vi "oa_Check DC Gap Input Data (N Channels).vi"(0 "even angle signals":cluster{"r0":dbl, "dr":dbl, "Y":dbl[]}[](array[cluster]) {"r0" format="%.2p"; "dr" format="%.2p"; "Y" format="%.2f"}, 1 "reset?":bool=TRUE, 5 "DC gap references [V]":dbl[](array[numeric]), 7 "averaging type in":enum16{"Linear", "Exponential"}(ring), 9 "window in":T1(ring), 11 "error in (no error)":errorcluster) -> (2 "reset DC ref?":bool, 3 "reset out?":bool, 4 "even angle signals":cluster{"r0":dbl, "dr":dbl, "Y":dbl[]}[](array[cluster]) {"r0" format="%.2p"; "dr" format="%.2p"; "Y" format="%.2f"}, 6 "DC gap reference [V]":dbl[](array[numeric]), 8 "averaging type":enum16{"Linear", "Exponential"}(ring), 10 "window":T1(ring), 15 "error out":errorcluster)   [LabVIEW 2017, in "SoundVib_RefDataProcess.lvlib"]
uses:
  <vilib>/addons/Sound and Vibration/Order Analysis/Referece Data Processing/SoundVib_RefDataProcess.lvlib
  <vilib>/addons/Sound and Vibration/Order Analysis/Resample Order Tracking/SubVIs/OAT Verify Resampled Signal (Multi Channels).vi
  <vilib>/addons/Sound and Vibration/Order Analysis/Resample Order Tracking/SoundVib_Resampling.lvlib
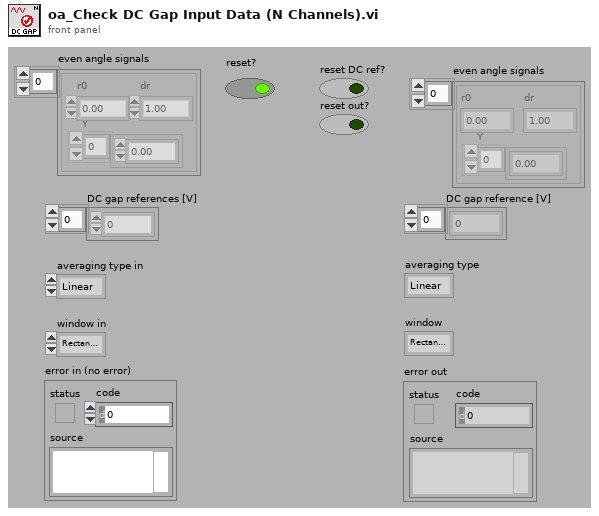
[diagram p1: front panel]
types:
  T1 = enum16{"Rectangular (none)", "Hanning", "Low side lobe"}
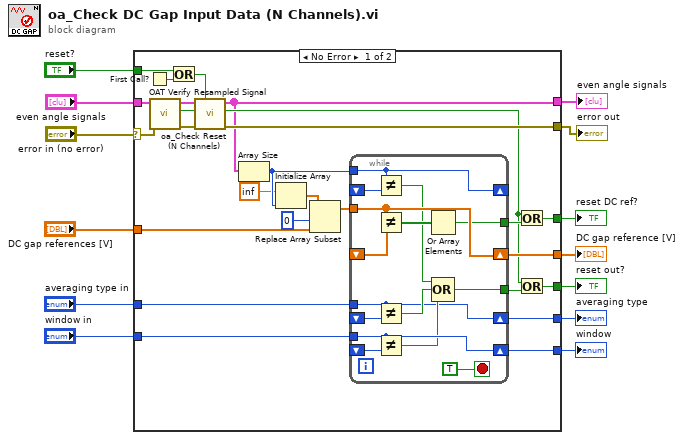
[diagram p0: block diagram]
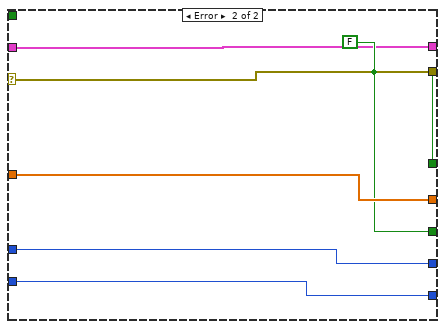
[diagram p2: hidden frame]
diagram:
  n1 = case shown="No Error" "error in (no error)" {
    selector: "error in (no error)" -> [w25 w58]
    tunnel: [w29 w56] -> w13
    tunnel: [w39 w59] -> w12
    tunnel: [w38 w60] -> w11
    tunnel: [w27 w56] -> w10
    tunnel: [w37 w57] -> w9
    tunnel: "DC gap references [V]" -> [w34 w57]
    tunnel: "window in" -> [w36 w59]
    tunnel: "averaging type in" -> [w35 w60]
    tunnel: "even angle signals" -> [w26 w55]
    tunnel: [w16 w58] -> w4
    tunnel: [w14 w55] -> w2
    tunnel: "reset?" -> [w31 _]
    frame No Error {
      n2 = First Call?() -> (First Call?: T/F=w32:bool)
      n3 = call-poly <vilib>:"OAT Verify Resampled Signal.vi"("error in (no error)"=w25, "resampled signal"=w26) -> ("error out"=w17:errorcluster, "empty signal"=w18:bool, "resampled signal out"=w20:cluster{"r0":dbl, "dr":dbl, "Y":dbl[]}[])  [unwired: 7 in]
      n4 = Or(x=w31, y=w32) -> (x .or. y?=w19:bool)
      n5 = call <vilib>:"oa_Check Reset (N Channels).vi"("reset?"=w19, "error in (no error)"=w17, "empty?"=w18, "resampled signal"=w20) -> ("error out"=w16:errorcluster, "reset?"=w15:bool, "resampled signal out"=w14:cluster{"r0":dbl, "dr":dbl, "Y":dbl[]}[])  [unwired: 5 in]
      n6 = Array Size(array=w14) -> (size(s)=w33:i32)
      n7 = Initialize Array(inf ("element"), w33) -> (w23:dbl[])
      n8 = Replace Array Subset(array=w23, new element=w34, index=0) -> (w22:dbl[])
      n9 = while {
        tunnel: w35 -> [w47]
        tunnel: w36 -> [w51]
        shift-right: [w47] -> w38
        shift-left: _ -> [w53]
        shift-right: [w51] -> w39
        shift-left: _ -> [w52]
        tunnel: [w48] -> w28
        tunnel: w22 -> [w44]
        shift-right: [w44] -> w37
        shift-left: _ -> [w46]
        tunnel: [w41] -> w30
        tunnel: w33 -> [w42]
        shift-right: [w42] -> _
        shift-left: _ -> [w43]
        stop <- TRUE stop-if-true
        n10 = Not Equal?(x=w42, y=w43) -> (x != y?=w40:bool)
        n11 = Not Equal?(x=w44, y=w46) -> (x != y?=w45:bool[])
        n12 = Not Equal?(x=w47, y=w53) -> (x != y?=w50:bool)
        n13 = Not Equal?(x=w51, y=w52) -> (x != y?=w49:bool)
        n14 = Or Array Elements(Boolean array=w45) -> (logical OR=w41:bool)
        n15 = Compound Arithmetic op=OR(w40, w50, w49) -> (w48:bool)
      }
      n16 = Or(x=w15, y=w30) -> (x .or. y?=w29:bool)
      n17 = Or(x=w15, y=w28) -> (x .or. y?=w27:bool)
    }
    frame Error {
      w56 = FALSE
    }
  }
  "reset DC ref?" <- w13
  "window" <- w12
  "averaging type" <- w11
  "reset out?" <- w10
  "DC gap reference [V]" <- w9
  "error out" <- w4
  "even angle signals" <- w2
